vi "Page_Dialog_Quit.vi"(6 "dialog info":T1, 8 "error in (no error)":errorcluster, 9 "data":variant, 10 "Target":refnum<vi>, 11 "Class in":refnum<class "Installer.lvclass">) -> (0 "error out":errorcluster, 3 "Class out":refnum<class "Installer.lvclass">)   [LabVIEW 2020, in "Installer.lvclass"]
uses:
  <vilib>/AppBuilder/IB_Classes/Installer/Installer.lvclass
  <vilib>/AppBuilder/IB_Classes/Installer/Installer.lvclass/Installer.ctl
  <resource>/Framework/Providers/Builds/Installer/CDK_sTypeDef_Languages.ctl
  <resource>/Framework/Providers/Builds/Installer/Pages/controls/IB_UI_Page_Dialog_Info_References.ctl
  <resource>/Framework/Providers/Common/provcom_BrowseProjectFile2.ctl
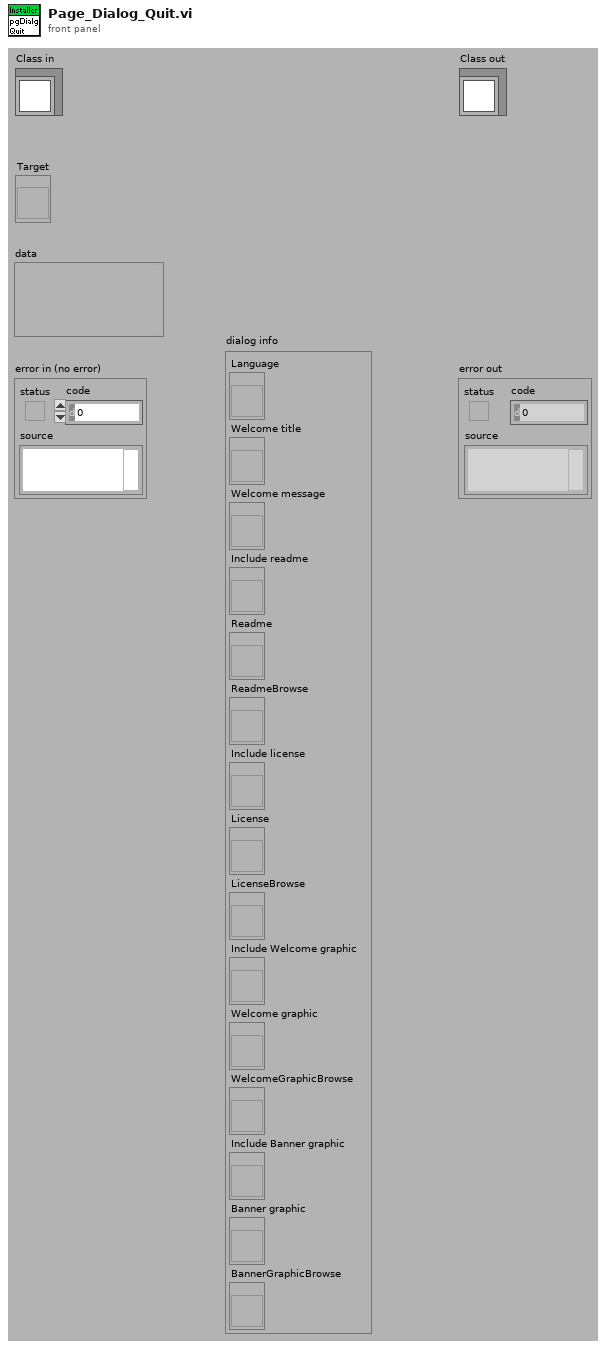
[diagram p1: front panel]
types:
  T1 = typedef "IB_UI_Page_Dialog_Info_References.ctl" = cluster{"Language":refnum<vi>, "Welcome title":refnum<vi>, "Welcome message":refnum<vi>, "Include readme":refnum<vi>, "Readme":refnum<vi>, "ReadmeBrowse":refnum<vi>, "Include license":refnum<vi>, "License":refnum<vi>, "LicenseBrowse":refnum<vi>, "Include Welcome graphic":refnum<vi>, "Welcome graphic":refnum<vi>, "WelcomeGraphicBrowse":refnum<vi>, "Include Banner graphic":refnum<vi>, "Banner graphic":refnum<vi>, "BannerGraphicBrowse":refnum<vi>}
  T2 = typedef "IB_Installer.ctl" = cluster{"Destination":refnum<class "IB_Destination.lvclass">[], "Source":refnum<class "IB_Source.lvclass">[], "buildObject":T3, "defaultDir":string, "platform":string, "author":string, "productName":string, "buildSpecName":string, "hide":bool, "requireLVDevSys":bool, "autoIncrement":bool, "includeError":bool, "readmeID":string, "buildLocation":path, "readmePath":path, "mediaSize":u16, "language":T4, "productVersion":T5, "preview":bool, "programmatic":bool, "progressBarEvents":T6, "userLog_Path":path, "shortcutAddresses":T8[], "EXE_Install Address":string, "EXE_Uninstall Address":string, "additional NIPaths":refnum<class "Dest_NI_NIPath.lvclass">[], "web service itemIDs":string[], "installerName":string}
  T3 = typedef "ItemRef.ctl" = u64
  T4 = typedef "CDK_sTypeDef_Languages.ctl" = u16
  T5 = typedef "CDK_sTypeDef_ProductVersion.ctl" = cluster{"Major":u8, "Minor":u8, "Update":u16}
  T6 = typedef "provcom_ProgressBar_Events.ctl" = cluster{"newJob":refnum<user-event>, "newItem":refnum<user-event>, "errorMsg":T7, "cancel":refnum<user-event>}
  T7 = typedef "mxLvBuildError.ctl" = refnum<user-event>
  T8 = typedef "CDK_sTypeDef_ShortcutAddress.ctl" = cluster{"file":string, "shortcut":string}
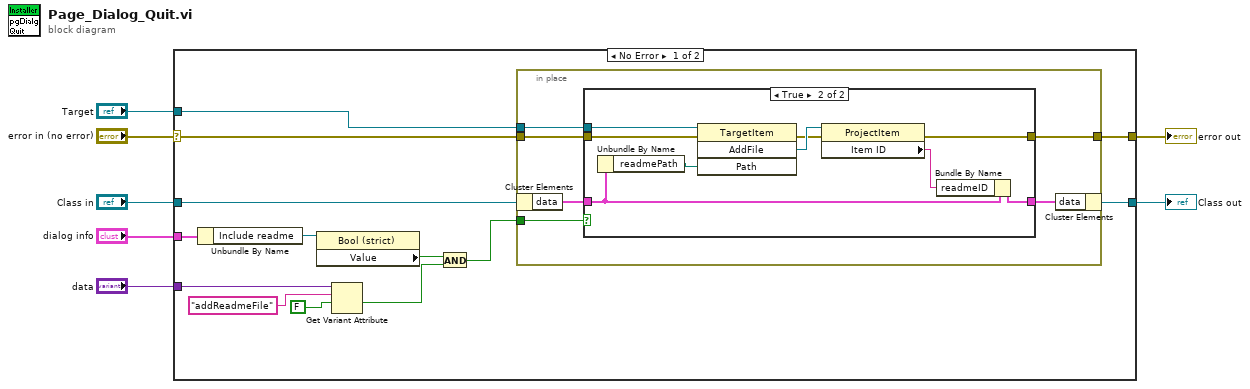
[diagram p0: block diagram]
diagram:
  n1 = case shown="No Error" "error in (no error)" {
    selector: "error in (no error)" -> [w9 w39]
    tunnel: [w8 w39] -> w6
    tunnel: [w13 w38] -> w4
    tunnel: "Class in" -> [w14 w38]
    tunnel: "dialog info" -> [w17 _]
    tunnel: "Target" -> [w15 _]
    tunnel: "data" -> [w19 _]
    frame No Error {
      n2 = Unbundle By Name(w17) -> ("Include readme"=w16:refnum<vi>)
      n3 = property class="Bool (strict)"(reference=w16) -> ("Value"=w12:bool)  [unwired: 1 in, 2 out]
      n4 = Get Variant Attribute(Variant=w19, name="addReadmeFile", default value (empty Variant)=FALSE) -> (value=w11:bool)  [unwired: 1 in, 3 out]
      n5 = And(x=w12, y=w11) -> (x .and. y?=w10:bool)
      n6 = in-place {
        in-place-border: w15 -> [w26]
        in-place-border: w10 -> [w23]
        in-place-border: [w22] -> w8
        in-place-border: w9 -> [w21]
        n7 = in-place-cluster #1(w14) -> ("data"=w25:T2)
        n8 = case shown="True" w23 {
          tunnel: w26 -> [_ w36]
          tunnel: w25 -> [w28 w34]
          tunnel: [w28 w32] -> w24
          tunnel: [w27 w30] -> w22
          tunnel: w21 -> [w27 w29]
          frame False {
          }
          frame True {
            n9 = Unbundle By Name(w34) -> ("readmePath"=w35:path)
            n10 = invoke class="TargetItem" method="AddFile"(reference=w36, error in=w29, "Path"=w35) -> (error out=w31:errorcluster, "AddFile"=w37:refnum<vi>)  [unwired: 1 in, 2 out]
            n11 = property class="ProjectItem"(reference=w37, error in=w31) -> (error out=w30:errorcluster, "Item ID"=w33:string)  [unwired: 1 out]
            n12 = Bundle By Name(cluster=w34, "readmeID"=w33) -> (w32:T2)
          }
        }
        n13 = in-place-cluster #1("data"=w24) -> (w13:refnum<class "Installer.lvclass">)
      }
    }
    frame Error {
    }
  }
  "error out" <- w6
  "Class out" <- w4
